vi "Test cCRD deserializer.vi"() -> ()   [LabVIEW 2012]
uses:
  CRDS/cCRDS/cCRDS.lvclass
  <userlib>/Serialization/JSON Serializer/JSON Serializer.lvclass
  <userlib>/Serialization/Formatter/Formatter.lvclass
  <userlib>/Serialization/JSON Deserializer/JSON Deserializer.lvclass
  <userlib>/Serialization/Formatter/Formatter.lvclass/Formatter.ctl
  <userlib>/Serialization/Serializer/Serializer.lvclass
  <userlib>/Serialization/Deserializer/Deserializer.lvclass
panel:
  out "error out":errorcluster
  out "specific class reference":refnum<class "cCRDS.lvclass">
  out "String":string
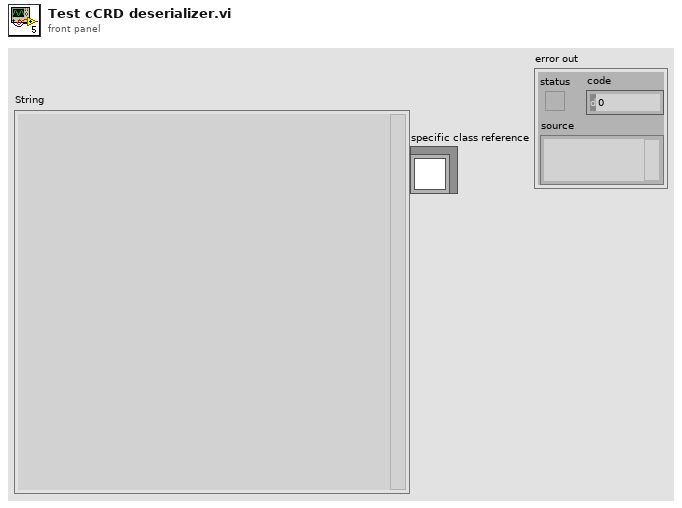
[diagram p1: front panel]
types:
  T1 = enum16{"No paths embedded", "One path with each object", "All paths with top object"}
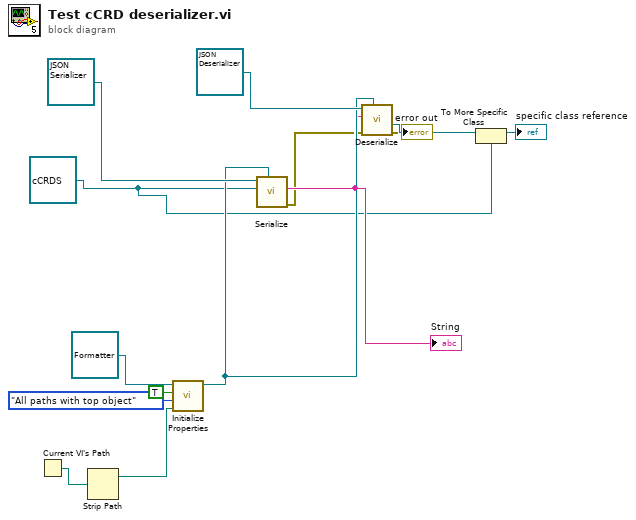
[diagram p0: block diagram]
diagram:
  w3 = refnum<class "cCRDS.lvclass"> refnum ("cPAS Server Library.lvlib:cCRDS")
  n1 = Current VI's Path() -> (path=w10:path)
  n2 = Strip Path(path=w10) -> (stripped path=w9:path)  [unwired: 1 out]
  n3 = call <userlib>:"Initialize Properties.vi"("Absolute Path For Dynamic Loading"=w9, "Path Embedding"=T1."All paths with top object", "Include all fields?"=TRUE, "Formatter in (Default Formatter)"=refnum<class "Formatter.lvclass"> refnum ("Formatter")) -> ("Formatter out"=w7:refnum<class "Formatter.lvclass">)  [unwired: 7 in]
  n4 = call <userlib>:"Serialize.vi"("Formatter (defaults)"=w7, "Serializable"=w3, "Serializer"=refnum<class "JSON Serializer.lvclass"> refnum ("JSON Serializer.lvclass")) -> ("error out"=w5:errorcluster, "String"=w6:string)  [unwired: 6 in, 1 out]
  "String" <- w6
  n5 = call <userlib>:"Deserialize.vi"("Formatter (defaults)"=w7, "error in (no error)"=w5, "String"=w6, "Deserializer"=refnum<class "JSON Deserializer.lvclass"> refnum ("JSON Deserializer.lvclass")) -> ("error out"=→"error out":errorcluster, "Serializable"=w4:refnum<class "Serializable.lvclass">)  [unwired: 5 in, 1 out]
  n6 = To More Specific Class(target class=w3, reference=w4) -> (specific class reference=→"specific class reference":refnum<class "cCRDS.lvclass">)  [unwired: 1 in, 1 out]
